vi "enable_chop_acquisition - multi-channel without switch.vi"() -> ()   [LabVIEW 2019]
doc: "This example demonstrates how to enable the Chop feature in a continuously acquire buffered voltage measurement using a DAQmx device.\n\nFor instructions on how to connect your signals to the DAQ device, refer to your device documentation."
uses:
  <vilib>/DAQmx/read.llb/DAQmx Read (Analog 2D DBL NChan NSamp).vi
  <vilib>/DAQmx/create/channels.llb/DAQmx Create Channel (AI-Voltage-Basic).vi
  <vilib>/DAQmx/configure/timing.llb/DAQmx Timing (Sample Clock).vi
  <vilib>/DAQmx/miscellaneous.llb/DAQmx Fill In Error Info.vi
  <resource>/objmgr/daqmx.rc
panel:
  out "Measurement 4":dbl[](graph)=[3.4836403218480996, 3.483638136505242, 3.4836380744758593, 3.4836399973867147, 3.48363957272402, 3.483638470509609, 3.4836413477186556, 3.483641190259454, 3.483640083273552, 3.4836384227946993, 3.4836387233986295, 3.483641190259454, 3.483640102359516, 3.4836416674085497, 3.4836375782408, 3.4836413095467282, 3.4836413906620742, 3.4836400594160972, 3.4836400498731153, 3.483636347196133, 3.483639954443296, 3.483642841195325, 3.4836401309884617, 3.4836414574629475, 3.4836386422832835, 3.4836394772942008, 3.4836418153247695, 3.483639109889397, 3.4836385182245184, 3.4836387711135393, 3.4836389142582678, 3.483641834410733]
  out "Measurement 3":dbl[](graph)=[3.4836386375117923, 3.483640994628325, 3.4836407226533406, 3.483637983817531, 3.4836385182245184, 3.483640464992829, 3.4836396013529654, 3.483639658610857, 3.4836407178818494, 3.483642440390085, 3.483640111902498, 3.483639095574924, 3.4836386375117923, 3.4836398303845315, 3.4836400451016245, 3.4836424737905216, 3.4836393961788543, 3.4836391671472886, 3.483642626478232, 3.4836386327403015, 3.4836413715761103, 3.483641977555462, 3.483638489595573, 3.483642082528263, 3.48364196801248, 3.4836381555912053, 3.4836421397861543, 3.483637983817531, 3.4836399114998775, 3.483638351222335, 3.4836398160700583, 3.48364056996563]
  out "Measurement 2":dbl[](graph)=[3.483637664127637, 3.483637754785965, 3.483640068959079, 3.4836405222507203, 3.4836408180831597, 3.4836389476587044, 3.483639944900314, 3.4836427219080512, 3.483637325351779, 3.483641051886216, 3.4836407226533406, 3.4836408705695603, 3.4836408610265783, 3.483641438376984, 3.48364226861641, 3.483638928572741, 3.483639439122273, 3.483638694769684, 3.4836409373704336, 3.4836372156074873, 3.4836419632409887, 3.4836414765489114, 3.483641209345418, 3.4836402025608257, 3.483640197789335, 3.48364156720724, 3.483641404976547, 3.483640278904681, 3.4836400498731153, 3.4836396108959473, 3.483639458208237, 3.483638861771867]
  out "error out":errorcluster
  in  "Total # of Channels":i32=128
  out "Elapsed Time (s)":dbl=0.3763147659992683 format="%#_3g"
  in  "Chop":bool=TRUE
  out "Measurement":dbl[](graph)=[3.4836374684965077, 3.4836391719187794, 3.4836404315923923, 3.4836401166739885, 3.4836401643888983, 3.4836389715161595, 3.48363727763687, 3.4836428077948884, 3.4836382653354976, 3.483639758812167, 3.483637998132004, 3.4836405127077383, 3.4836414479199656, 3.4836388665433584, 3.4836398399275135, 3.483639849470495, 3.4836408228546505, 3.483641948926516, 3.483640484078793, 3.483641228431382, 3.483639854241986, 3.4836387567990665, 3.48363837985128, 3.4836416101506584, 3.4836412713748004, 3.483641705580477, 3.4836384323376812, 3.4836378359013116, 3.4836406749384308, 3.4836385086815365, 3.483639429579291, 3.483644706848289]
  in  "Terminal Configuration":i32(ring)=10106 items=["default"=-1, "RSE"=10083, "NRSE"=10078, "Differential"=10106, "Pseudodifferential"=12529]
  in  "Max Voltage":dbl=10.0
  in  "Min Voltage":dbl=-10.0
  in  "Physical Channel":tag="4309/ai0:3"
  # "DAQmx Settings"
  # "On (T)"
  # "Off (F)"
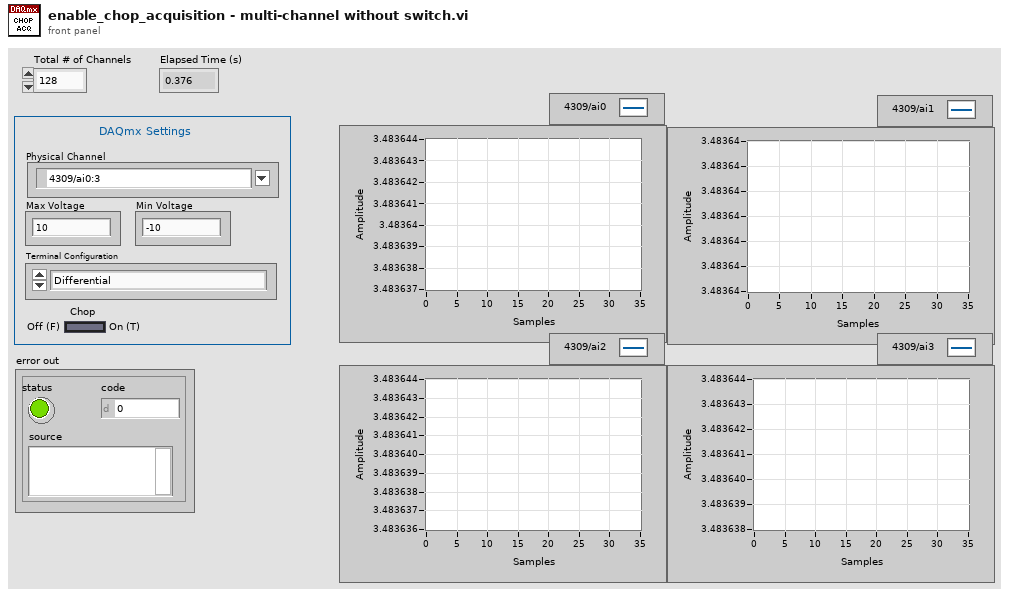
[diagram p1: front panel]
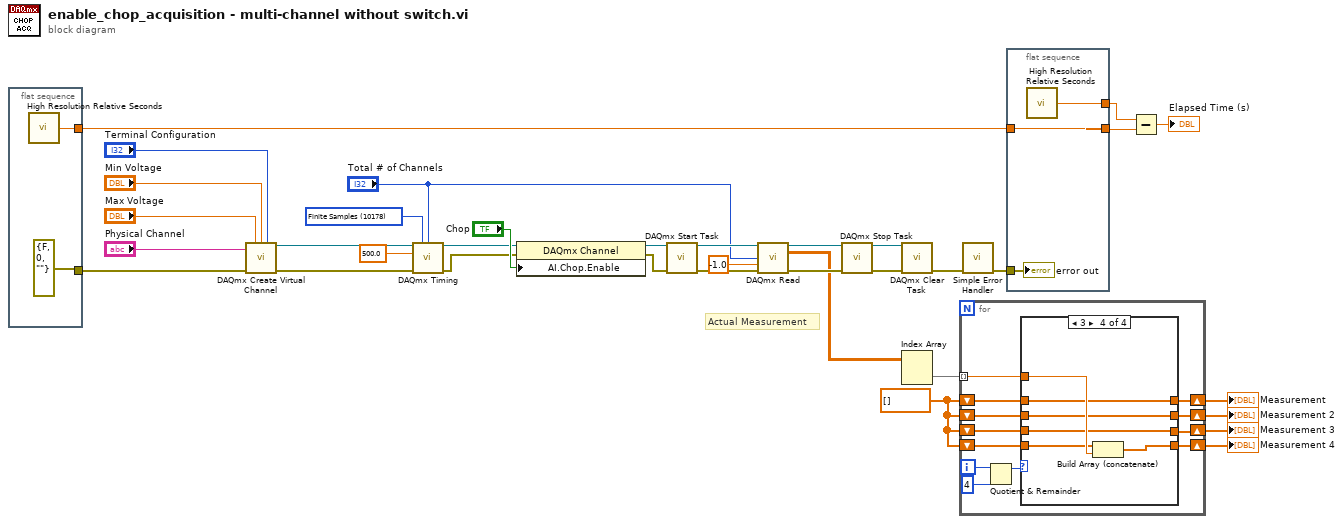
[diagram p0: block diagram]
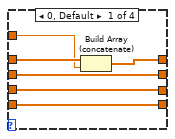
[diagram p2: hidden frame]
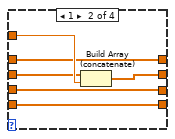
[diagram p3: hidden frame]
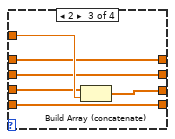
[diagram p4: hidden frame]
diagram:
  w6 = dbl[] [] ("History Data")
  w14 = 10178 items=["Finite Samples"=10178, "Continuous Samples"=10123, "Hardware Timed Single Point"=12522] ("sample mode")
  # "Actual Measurement"
  n1 = flat-sequence {
    tunnel: [w37] -> w26
    tunnel: [errorcluster {"status"=FALSE, "code"=0, "source"=""} ("error out")] -> w4
    frame #0 {
      n2 = call <vilib>:"High Resolution Relative Seconds.vi"() -> ("relative seconds"=w37:dbl)
    }
  }
  n3 = call-poly <vilib>:"DAQmx Create Virtual Channel.vi"("maximum value"="Max Voltage", "minimum value"="Min Voltage", "input terminal configuration"="Terminal Configuration", "physical channels"="Physical Channel", "error in"=w4) -> ("task out"=w19:refnum<k21>, "error out"=w22:errorcluster)  [unwired: 9 in]
  n4 = call-poly <vilib>:"DAQmx Timing.vi"("task/channels in"=w19, "sample mode"=w14, "samples per channel"="Total # of Channels", "rate"=500.0, "error in"=w22) -> ("task out"=w20:refnum<k21>, "error out"=w21:errorcluster)  [unwired: 9 in]
  n5 = property class="DAQmx Channel"(reference=w20, error in=w21, "AI.Chop.Enable"="Chop") -> (reference out=w18:refnum<k21>, error out=w17:errorcluster)
  n6 = call <vilib>:"DAQmx Start Task.vi"("task/channels in"=w18, "error in"=w17) -> ("task out"=w16:refnum<k21>, "error out"=w5:errorcluster)  [unwired: 12 in]
  n7 = call-poly <vilib>:"DAQmx Read.vi"("task/channels in"=w16, "number of samples per channel"="Total # of Channels", "timeout"=-1.0, "error in"=w5) -> ("task out"=w12:refnum<k21>, "data"=w2:dbl[][], "error out"=w13:errorcluster)  [unwired: 9 in]
  n8 = call <vilib>:"DAQmx Stop Task.vi"("task/channels in"=w12, "error in"=w13) -> ("task out"=w30:refnum<k21>, "error out"=w31:errorcluster)  [unwired: 12 in]
  n9 = call <vilib>:"DAQmx Clear Task.vi"("task in"=w30, "error in"=w31) -> ("error out"=w28:errorcluster)  [unwired: 13 in]
  n10 = Index Array(array=w2) -> (element=w11:dbl[])  [unwired: 2 in]
  n11 = for {
    tunnel: w11 -> [w46] mode=indexing
    shift-right: [w44] -> w10
    shift-left: w6 -> [w45]
    shift-right: [w43] -> w9
    shift-left: w6 -> [w42]
    shift-right: [w41] -> w8
    shift-left: w6 -> [w40]
    shift-right: [w39] -> w7
    shift-left: w6 -> [w38]
    i -> [w49]
    n12 = Quotient & Remainder(x=w49, y=4) -> (x-y*floor(x/y)=w47:i32)  [unwired: 1 out]
    n13 = case shown="3" w47 {
      tunnel: w46 -> [w53 w61 w67 w73]
      tunnel: w45 -> [w54 w58 w64 w70]
      tunnel: [w55 w58 w64 w70] -> w44
      tunnel: [w52 w60 w63 w69] -> w43
      tunnel: w42 -> [w52 w59 w63 w69]
      tunnel: [w51 w57 w66 w68] -> w41
      tunnel: w40 -> [w51 w57 w65 w68]
      tunnel: [w50 w56 w62 w72] -> w39
      tunnel: w38 -> [w50 w56 w62 w71]
      frame 0, Default {
        n14 = Build Array (concatenate)(w54, w53) -> (w55:dbl[])
      }
      frame 1 {
        n15 = Build Array (concatenate)(w59, w61) -> (w60:dbl[])
      }
      frame 2 {
        n16 = Build Array (concatenate)(w65, w67) -> (w66:dbl[])
      }
      frame 3 {
        n17 = Build Array (concatenate)(w71, w73) -> (w72:dbl[])
      }
    }
  }
  "Measurement" <- w10
  "Measurement 2" <- w9
  "Measurement 3" <- w8
  "Measurement 4" <- w7
  n18 = call <vilib>:"Simple Error Handler.vi"("error in (no error)"=w28) -> ("error out"=w27:errorcluster)  [unwired: 1 in, 7 out]
  n19 = flat-sequence {
    tunnel: w27 -> [w74]
    tunnel: [w76] -> w25
    tunnel: w26 -> [w75]
    tunnel: [w75] -> w24
    frame #0 {
      n20 = call <vilib>:"High Resolution Relative Seconds.vi"() -> ("relative seconds"=w76:dbl)
      "error out" <- w74
    }
  }
  n21 = Subtract(x=w25, y=w24) -> (x-y=→"Elapsed Time (s)":dbl)
